vi "com attempt3.vi"() -> ()   [LabVIEW 2020]
uses:
  Program Files (x86)/National Instruments/LabVIEW 2020/examples/Instrument IO/Serial/support/Serial - Settings.ctl
  <vilib>/Instr/_visa.llb/VISA Configure Serial Port (Instr).vi
panel:
  out "*(type *) &x":i32 format="%x"
  in  "Numeric":i32 format="%x"
  out "Array":cluster{"send":i32, "return":string}[](array[cluster])
  out "Read 2":bool
  out "Serial Settings:Number of Bytes at Serial Port":u32
  out "Response":string
  out "Command":string="*IDN?"
  in  "Stop":bool
  in  "Write":bool
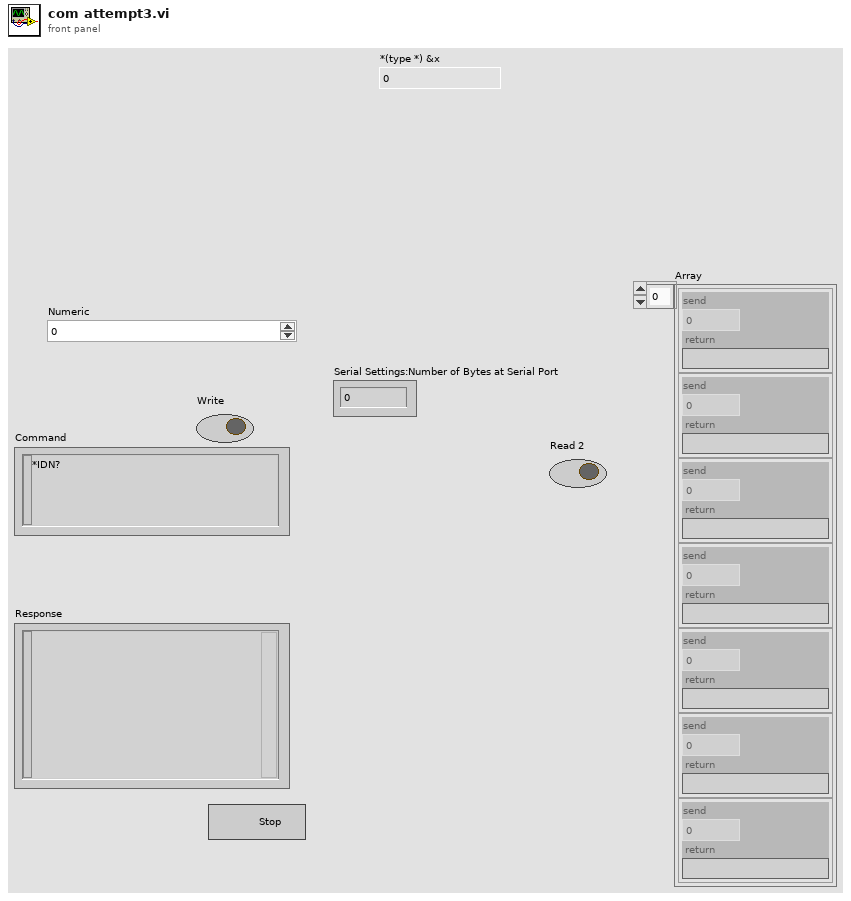
[diagram p1: front panel]
types:
  T1 = typedef "Serial - Settings.ctl" = cluster{"baud rate":u32, "data bits":u16, "parity":enum16{"None", "Odd", "Even", "Mark", "Space"}, "stop bits":u16, "flow control":u16}
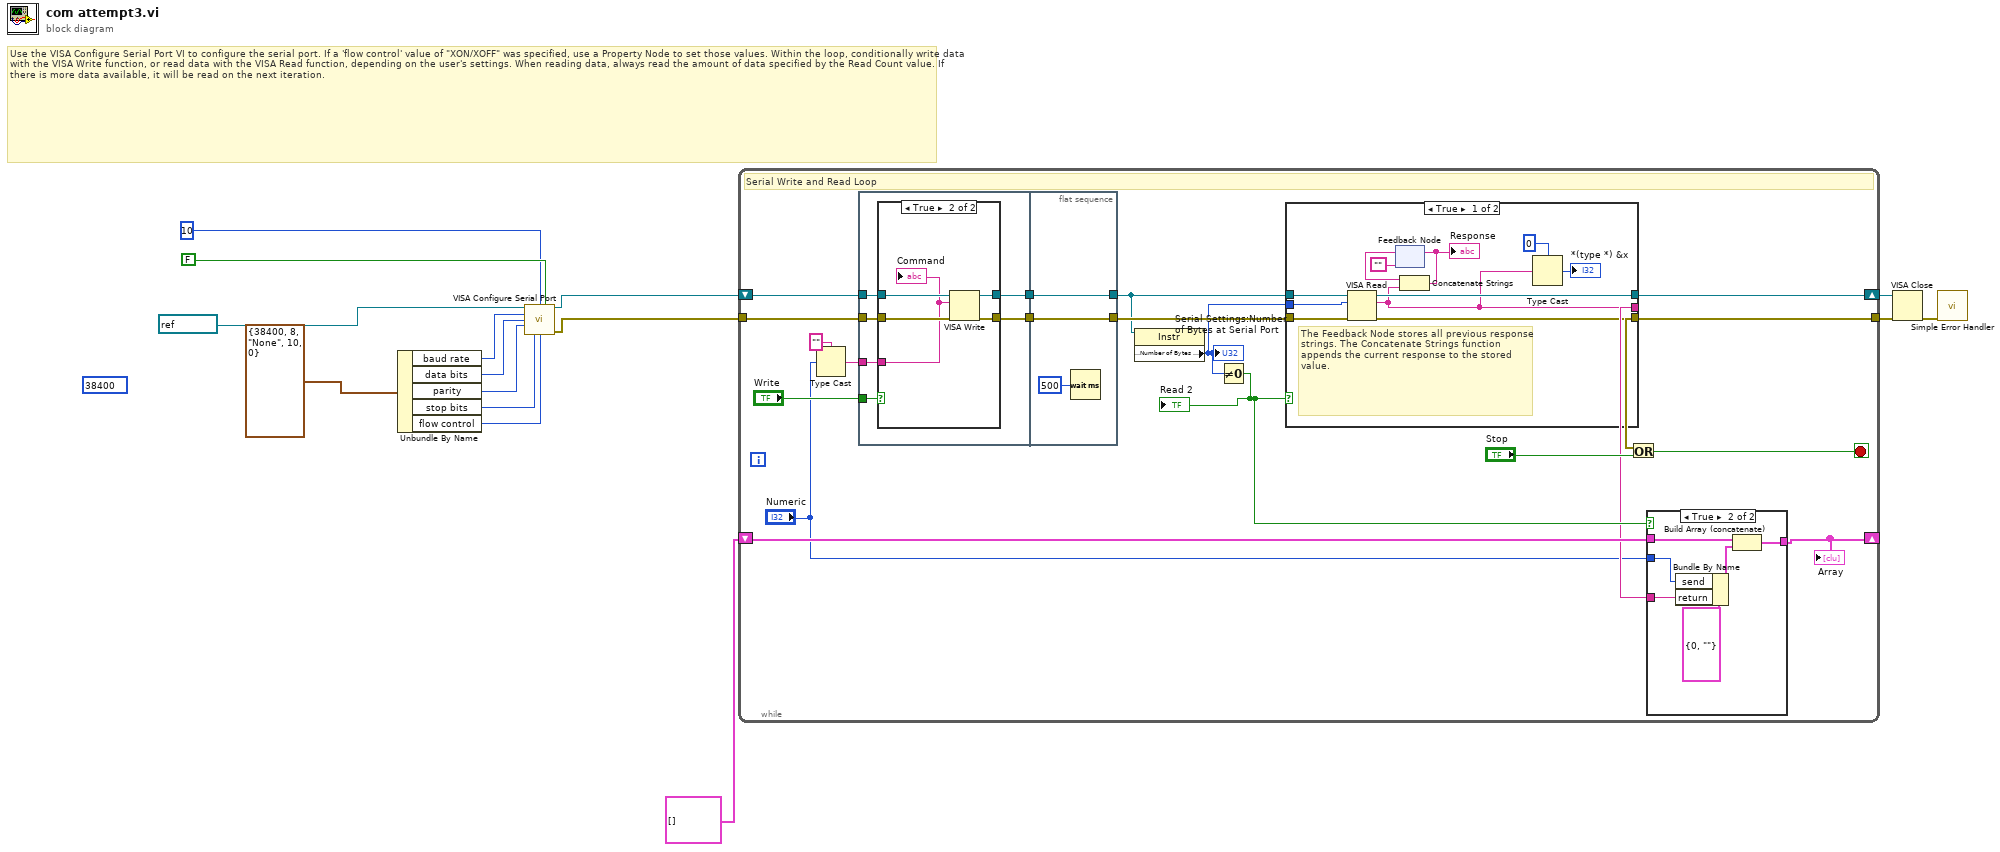
[diagram p0: block diagram]
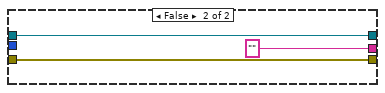
[diagram p4: hidden frame]
diagram:
  (unwired) u32 38400 items=["75"=75, "110"=110, "134"=134, "150"=150, "300"=300, "600"=600, "1200"=1200, "1800"=1800, "2400"=2400, "4800"=4800, "7200"=7200, "9600"=9600, "14400"=14400, "19200"=19200, "28800"=28800, "38400"=38400, "56000"=56000, "57600"=57600, "115200"=115200, "128000"=128000, "230400"=230400] ("baud rate")
  # "Use the VISA Configure Serial Port VI to configure the serial port. If a 'flow control' value of \"XON/XOFF\" was specified, use a Property Node to set those values. Within the loop, conditionally write data with the VISA Write function, or read data with the VISA Read function, depending on the user's settings. When reading data, always read the amount of data specified by the Read Count value. If there is more data available, it will be read on the next iteration."
  n1 = Unbundle By Name(T1 {"baud rate"=38400, "data bits"=8, "parity"=enum."None", "stop bits"=10, "flow control"=0} ("Serial Settings")) -> ("baud rate"=w7:u32, "data bits"=w8:u16, "parity"=w9:enum16{"None", "Odd", "Even", "Mark", "Space"}, "stop bits"=w10:u16, "flow control"=w4:u16)
  n2 = call-poly "VISA Configure Serial Port"("VISA resource name"=refnum<visa-resource-name> "COM4", "termination char\n(0xA = '\\n' = LF)"=u8 10 ("Termination Character"), "Enable Termination\nChar (T)"=FALSE ("End Read on Termination Character?"), "baud rate (9600)"=w7, "data bits (8)"=w8, "parity (0:none)"=w9, "stop bits (10: 1 bit)"=w10, "flow control (0:none)"=w4) -> ("VISA resource name out"=w2:refnum<visa-resource-name>, "error out"=w1:errorcluster)  [unwired: 2 in, 4 out]
  n3 = while {
    shift-right: [w34] -> w13
    shift-left: w2 -> [w33]
    tunnel: w1 -> [w32]
    tunnel: [w29] -> w14
    shift-right: [w22] -> _
    shift-left: cluster{i32, "read buffer":string}[] [] -> [w20]
    stop <- w30 stop-if-true
    # "Serial Write and Read Loop"
    n4 = Type Cast(type="", x="Numeric") -> (*(type *) &x=w25:string)
    n5 = flat-sequence {
      tunnel: w33 -> [w47]
      tunnel: w32 -> [w46]
      tunnel: "Write" -> [w43]
      tunnel: w25 -> [w42]
      tunnel: [w45] -> w24
      tunnel: [w44] -> w23
      tunnel: [w56] -> w31
      tunnel: [w57] -> w19
      tunnel: w24 -> [w57]
      tunnel: w23 -> [w56]
      frame #0 {
        n6 = case shown="True" w43 {
          tunnel: w47 -> [w49 w54]
          tunnel: w46 -> [w48 w53]
          tunnel: [w49 w52] -> w45
          tunnel: [w48 w51] -> w44
          tunnel: w42 -> [_ w50]
          frame False {
          }
          frame True {
            n7 = VISA Write(VISA resource name=w54, write buffer=w50, error in (no error)=w53) -> (VISA resource name out=w52:refnum<visa-resource-name>, error out=w51:errorcluster)  [unwired: 1 out]
            "Command" <- w50
          }
        }
      }
      frame #1 {
        n8 = Wait (ms)(milliseconds to wait=u32 500) -> ()  [unwired: 1 out]
      }
    }
    n9 = property class="Instr"(reference=w19) -> ("Serial Settings:Number of Bytes at Serial Port"=w18:u32)  [unwired: 1 in, 2 out]
    "Serial Settings:Number of Bytes at Serial Port" <- w18
    n10 = Not Equal To 0?(x=w18) -> (x != 0?=w21:bool)
    "Read 2" <- w21
    n11 = case shown="True" w21 {
      tunnel: [w66 w71] -> w34
      tunnel: w19 -> [w68 w71]
      tunnel: [w65 w70] -> w29
      tunnel: w31 -> [w67 w70]
      tunnel: w18 -> [w61 _]
      tunnel: [w60 "" ("read buffer")] -> w17
      frame True {
        # "The Feedback Node stores all previous response strings. The Concatenate Strings function appends the current response to the stored value."
        n12 = VISA Read(VISA resource name=w68, byte count=w61, error in (no error)=w67) -> (VISA resource name out=w66:refnum<visa-resource-name>, read buffer=w60:string, error out=w65:errorcluster)  [unwired: 1 out]
        n13 = feedback #1("") -> (w64:string)
        n14 = Concatenate Strings(w64, w60) -> (w63:string)
        "Response" <- w63
        n15 = feedback-in #1(w63) -> ()
        n16 = Type Cast(type=0 ("Numeric"), x=w60) -> (*(type *) &x=→"*(type *) &x":i32)
      }
      frame False {
      }
    }
    n17 = Or(x=w29, y="Stop") -> (x .or. y?=w30:bool)
    n18 = case shown="True" w21 {
      tunnel: "Numeric" -> [_ w37]
      tunnel: [w35 w41] -> w22
      tunnel: w20 -> [w35 w40]
      tunnel: w17 -> [_ w36]
      frame False {
      }
      frame True {
        n19 = Bundle By Name(cluster=cluster{"send":i32, "return":string} {"send"=0, "return"=""} ("Cluster"), "send"=w37, "return"=w36) -> (w38:cluster{"send":i32, "return":string})
        n20 = Build Array (concatenate)(w40, w38) -> (w41:cluster{"send":i32, "return":string}[])
      }
    }
    "Array" <- w22
  }
  n21 = VISA Close(VISA resource name=w13, error in (no error)=w14) -> (error out=w15:errorcluster)
  n22 = call <vilib>:"Simple Error Handler.vi"("error in (no error)"=w15) -> ()  [unwired: 1 in, 8 out]
